vi "Extract MultiSourceFrame Data.vi"(7 "Data Type Enabled?":bool, 8 "error in (no error)":errorcluster, 9 "Frame Data Type":i32, 10 "Frame Data in":variant, 11 "MultiSourceFrame Reference in":refnum<k24>) -> (0 "error out":errorcluster, 3 "Frame Data out":variant)   [LabVIEW 2014]
uses:
  Microsoft.Kinect
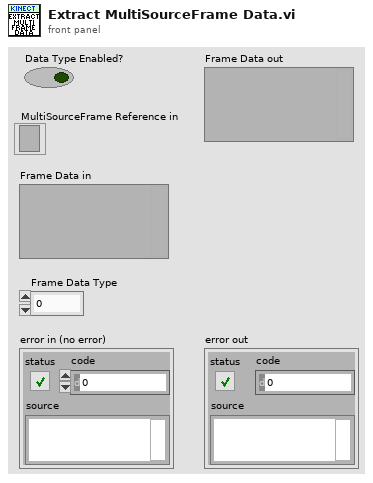
[diagram p1: front panel]
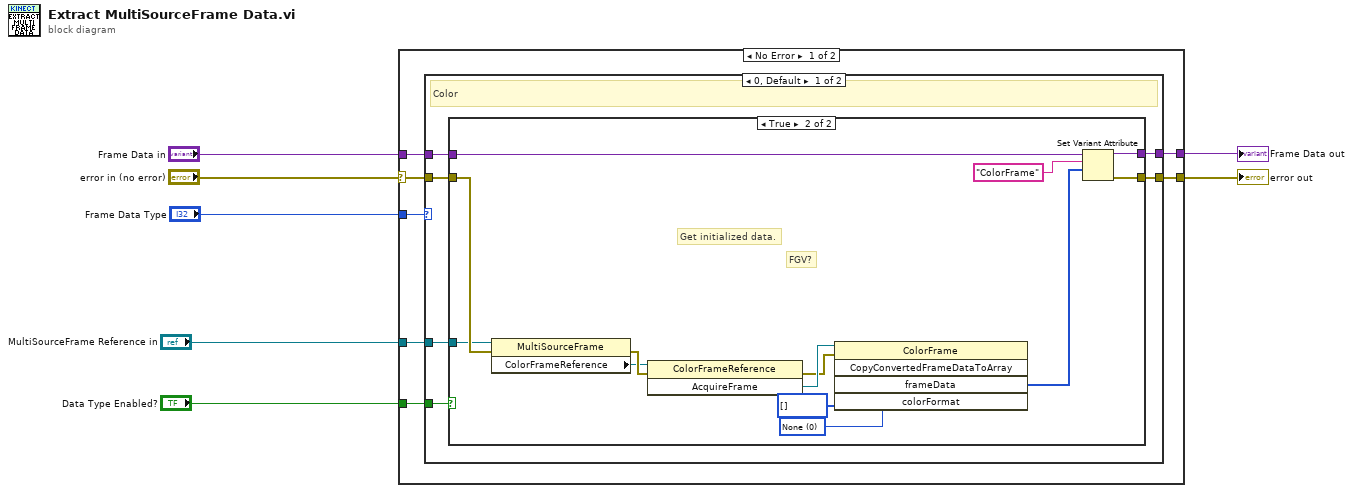
[diagram p0: block diagram]
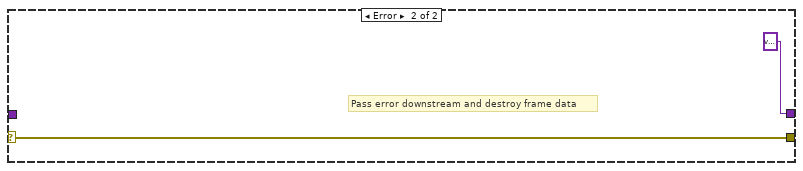
[diagram p4: hidden frame]
diagram:
  n1 = case shown="No Error" "error in (no error)" {
    selector: "error in (no error)" -> [w9 w39]
    tunnel: [w14 variant] -> w1
    tunnel: [w13 w39] -> w2
    tunnel: "Frame Data in" -> [w10 _]
    tunnel: "Frame Data Type" -> [w12 _]
    tunnel: "Data Type Enabled?" -> [w11 _]
    tunnel: "MultiSourceFrame Reference in" -> [w8 _]
    frame No Error {
      n2 = case shown="0, Default" w12 {
        tunnel: [w20 w37] -> w14
        tunnel: [w19 w36] -> w13
        tunnel: w11 -> [w18 _]
        tunnel: w10 -> [w17 w37]
        tunnel: w9 -> [w16 w36]
        tunnel: w8 -> [w15 _]
        frame 0, Default {
          # "Color"
          n3 = case shown="True" w18 {
            tunnel: [w22 w35] -> w20
            tunnel: [w21 w34] -> w19
            tunnel: w17 -> [w22 w31]
            tunnel: w16 -> [w21 w32]
            tunnel: w15 -> [_ w24]
            frame False {
            }
            frame True {
              w25 = 0 items=["None", "Rgba", "Yuv", "Bgra", "Bayer", "Yuy2"] ("colorFormat")
              # "FGV?"
              # "Get initialized data."
              n4 = property class="MultiSourceFrame"(reference=w24, error in=w32) -> (error out=w30:errorcluster, "ColorFrameReference"=w23:refnum<k24>)  [unwired: 1 out]
              n5 = invoke class="ColorFrameReference" method="AcquireFrame"(reference=w23, error in=w30) -> (error out=w27:errorcluster, "AcquireFrame"=w29:refnum<k24>)  [unwired: 1 in, 1 out]
              n6 = invoke class="ColorFrame" method="CopyConvertedFrameDataToArray"(reference=w29, error in=w27, "frameData"=u8[] [], "colorFormat"=w25) -> ("frameData"=w28:u8[])  [unwired: 1 in, 4 out]
              n7 = Set Variant Attribute(Variant=w31, name="ColorFrame", value=w28) -> (Variant out=w35:variant, error out=w34:errorcluster)  [unwired: 1 in, 1 out]
            }
          }
        }
        frame 1 {
          # "Infrared"
        }
      }
    }
    frame Error {
      # "Pass error downstream and destroy frame data"
    }
  }
  "error out" <- w2
  "Frame Data out" <- w1
